vi "mono1stgf.vi"() -> ()   [LabVIEW 2010]
panel:
  in  "Tab Control":enum32{"Page 1", "Page 2"}(tab)
  in  "Initial Wavelength (nm)":dbl=476.2
  in  "Parallel Port Address":i16=888 format="%.0x"
  in  "Stop Wavelenth (nm)":dbl=476.0
  in  "Ring":u16(ring) items=["Up", "Down"]
  in  "Number of steps":i32=1
  # "Set Up"
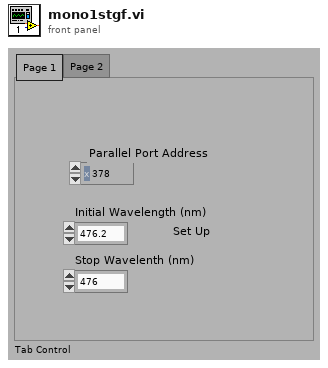
[diagram p1: front panel]
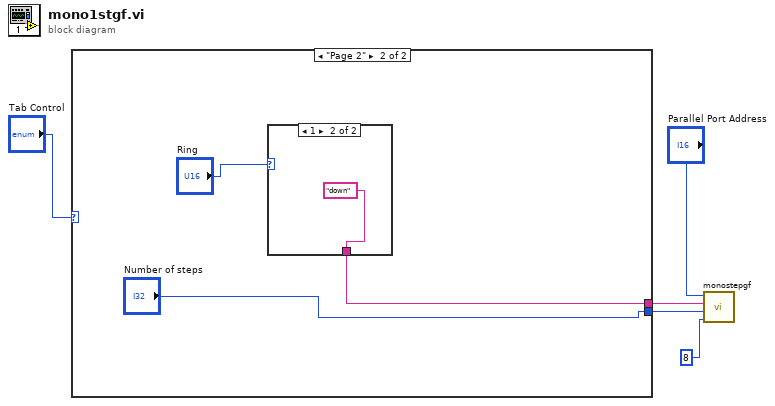
[diagram p0: block diagram]
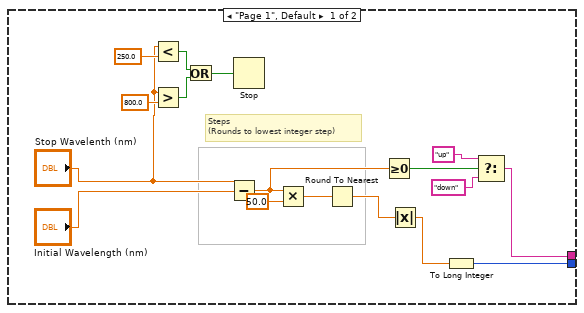
[diagram p2: hidden frame]
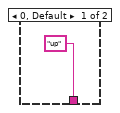
[diagram p3: hidden frame]
diagram:
  n1 = case shown="\"Page 2\"" "Tab Control" {
    tunnel: [w15 w23] -> w5
    tunnel: [w6 "Number of steps"] -> w4
    frame "Page 1", Default {
      # "Steps \n(Rounds to lowest integer step)"
      n2 = Less?(x="Stop Wavelenth (nm)", y=250.0) -> (x < y?=w11:bool)
      n3 = Greater?(x="Stop Wavelenth (nm)", y=800.0) -> (0:w10:bool)
      n4 = Or(x=w11, y=w10) -> (x .or. y?=w9:bool)
      n5 = Subtract(x="Stop Wavelenth (nm)", y="Initial Wavelength (nm)") -> (x-y=w19:dbl)
      n6 = Stop(stop? (T)=w9) -> ()
      n7 = Multiply(x=w19, y=50.0) -> (x*y=w20:dbl)
      n8 = Round To Nearest(number=w20) -> (nearest integer value=w8:dbl)
      n9 = Greater Or Equal To 0?(x=w19) -> (x >= 0?=w18:bool)
      n10 = Absolute Value(x=w8) -> (abs(x)=w7:dbl)
      n11 = To Long Integer(number=w7) -> (32bit integer=w6:i32)
      n12 = Select(t="up", s=w18, f="down") -> (s? t:f=w15:string)
    }
    frame "Page 2" {
      n13 = case shown="1" "Ring" {
        tunnel: ["up" "down"] -> w23
        frame 0, Default {
        }
        frame 1 {
        }
      }
    }
  }
  n14 = call "monostepgf.vi"("Wait Between Steps(ms)"=u32 8, "Steps"=w4, "Direction"=w5, "address"="Parallel Port Address") -> ()
